vi "GetGain.vi"(8 "error in (no error)":errorcluster, 11 "Camera_Prime95B in":refnum<class "Camera_Prime95B.lvclass">) -> (0 "error out":errorcluster, 2 "Setting.Gain":i32, 3 "Camera_Prime95B out":refnum<class "Camera_Prime95B.lvclass">)   [LabVIEW 2020, in "Camera_Prime95B.lvlib" / "Camera_Prime95B.lvclass"]
uses:
  Camera_Prime95B.lvclass
  Camera_Prime95B.lvclass/Camera_Prime95B.ctl
  E:/Development/DevHardSoftware/MicroscopyFramework/Model/Hardware Layer/Real Hardware/Camera_Prime95B/Camera_Prime95B/Dependencies/PVCamNET.dll
  Dependencies/PVCamNET.dll
  Hardware Abstraction Layer/Component/Camera/Camera/Camera.lvclass
panel:
  out "Name":string
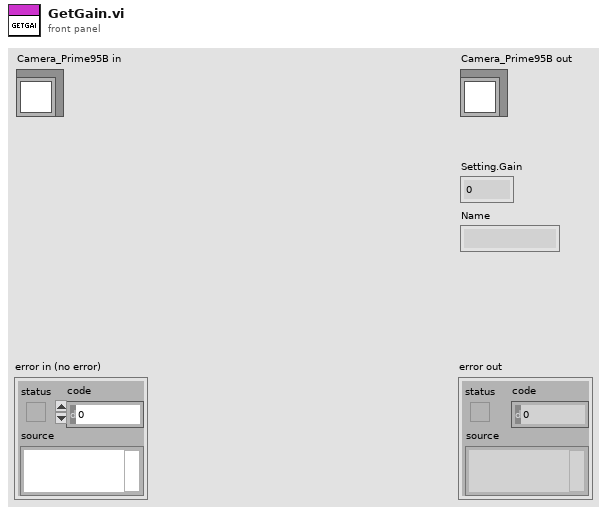
[diagram p1: front panel]
types:
  T1 = typedef "Device.lvlib/DeviceStatus.ctl" = i32
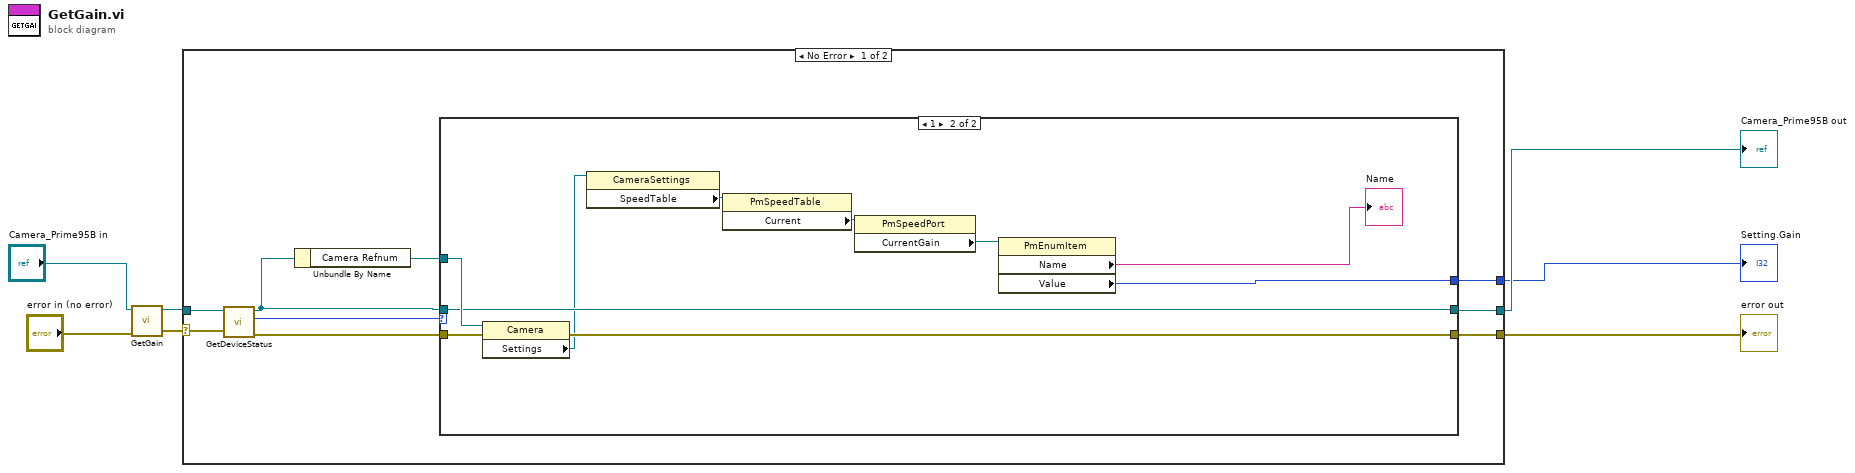
[diagram p0: block diagram]
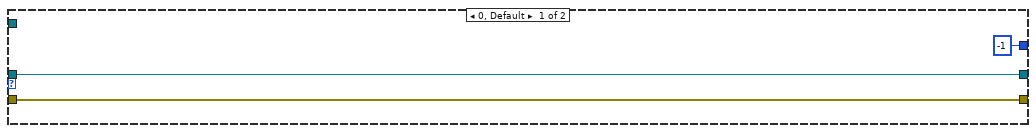
[diagram p2: hidden frame]
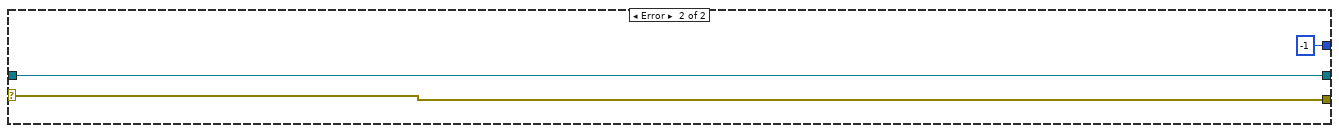
[diagram p3: hidden frame]
diagram:
  n1 = call-parent "GetGain.vi"("error in (no error)"="error in (no error)", "Camera in"="Camera_Prime95B in") -> ("error out"=w1:errorcluster, "Camera out"=w5:refnum<class "Camera_Prime95B.lvclass">)  [unwired: 7 in, 1 out]
  n2 = case shown="No Error" w1 {
    selector: w1 -> [w15 w32]
    tunnel: [w16 w32] -> w3
    tunnel: [w10 w31] -> w4
    tunnel: w5 -> [w9 w31]
    tunnel: [w8 -1 ("Value")] -> w2
    frame No Error {
      n3 = call-dynamic "GetDeviceStatus.vi"("error in (no error)"=w15, "Camera_Prime95B in"=w9) -> ("error out"=w13:errorcluster, "Status"=w14:T1, "Camera_Prime95B out"=w11:refnum<class "Camera_Prime95B.lvclass">)  [unwired: 7 in]
      n4 = Unbundle By Name(w11) -> ("Camera Refnum"=w12:refnum<k24>)
      n5 = case shown="1" w14 {
        tunnel: [w18 w29] -> w16
        tunnel: w12 -> [_ w28]
        tunnel: w13 -> [w18 w27]
        tunnel: w11 -> [w19 w26]
        tunnel: [w19 w26] -> w10
        tunnel: [-1 ("Value") w20] -> w8
        frame 0, Default {
        }
        frame 1 {
          n6 = property class="Camera"(reference=w28, error in=w27) -> (error out=w29:errorcluster, "Settings"=w23:refnum<k24>)  [unwired: 1 out]
          n7 = property class="CameraSettings"(reference=w23) -> ("SpeedTable"=w25:refnum<k24>)  [unwired: 1 in, 2 out]
          n8 = property class="PmSpeedTable"(reference=w25) -> ("Current"=w24:refnum<k24>)  [unwired: 1 in, 2 out]
          n9 = property class="PmSpeedPort"(reference=w24) -> ("CurrentGain"=w21:refnum<k24>)  [unwired: 1 in, 2 out]
          n10 = property class="PmEnumItem"(reference=w21) -> ("Name"=→"Name":string, "Value"=w20:i32)  [unwired: 1 in, 2 out]
        }
      }
    }
    frame Error {
    }
  }
  "error out" <- w3
  "Camera_Prime95B out" <- w4
  "Setting.Gain" <- w2
